vi "Initialization.vi"(3 "AdapterModuleRequired":bool=TRUE) -> (0 "InitDone":bool, 1 "IO Module ID":T1 {"InsertedIOModule ID" format="%x"; "Expected IO Module ID" format="%x"})   [LabVIEW 2013, in "IRIO.lvlib"]
uses:
  IRIO.lvlib
  <vilib>/eio/EIONode/EIONode.xnode
  <vilib>/rvi/eio/common/nirviEmuTemplateMethod_errors.vi
panel:
  out "IO Module IO Enabled":bool
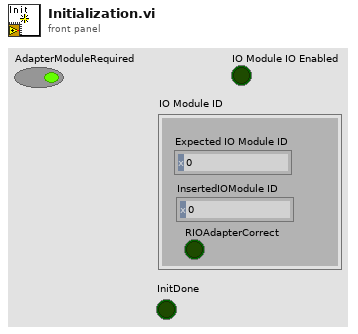
[diagram p1: front panel]
types:
  T1 = cluster{"Expected IO Module ID":u32, "InsertedIOModule ID":u32, "RIOAdapterCorrect":bool}
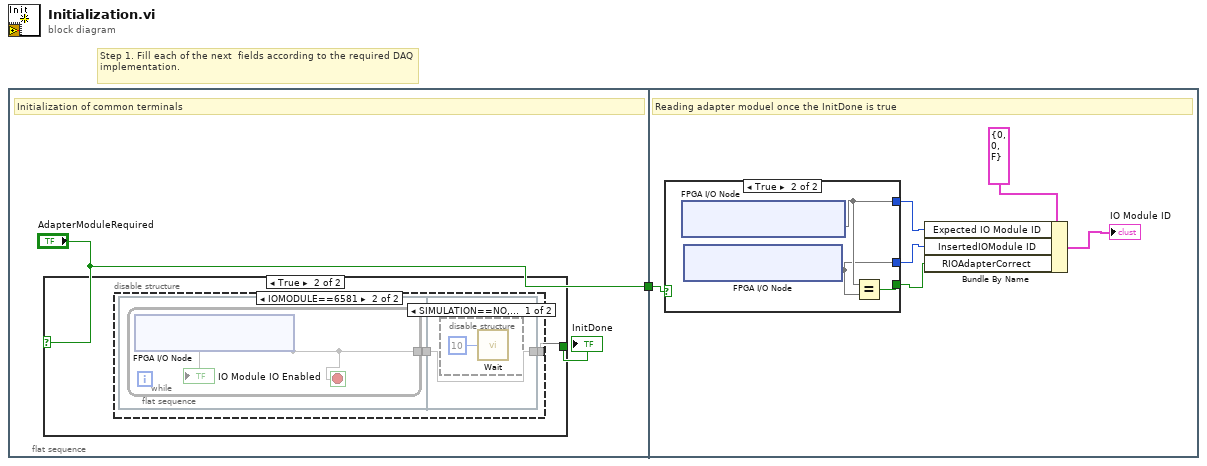
[diagram p0: block diagram]
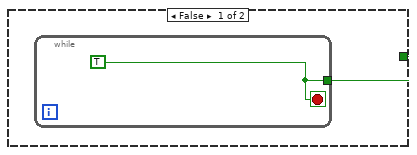
[diagram p2: hidden frame]
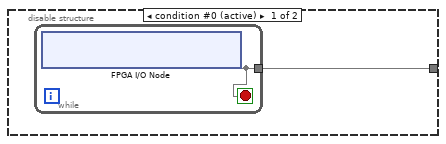
[diagram p3: hidden frame]
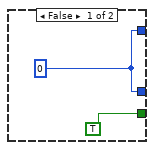
[diagram p5: hidden frame]
diagram:
  # "Step 1. Fill each of the next  fields according to the required DAQ implementation."
  n1 = flat-sequence {
    tunnel: ["AdapterModuleRequired"] -> w1
    tunnel: w1 -> [w20]
    frame #0 {
      # "Initialization of common terminals"
      n2 = case shown="True" "AdapterModuleRequired" {
        tunnel: [w4 w6] -> w3
        frame False {
          n3 = while {
            tunnel: [w5] -> w4
            stop <- w5 stop-if-true
            w5 = TRUE
          }
        }
        frame True {
          n4 = disable-structure shown="IOMODULE==6581" {
            disable-tunnel: [w7 w10] -> w6
            frame condition #0 (active) {
              n5 = while {
                tunnel: [w8] -> w7
                stop <- w8 stop-if-true
                n6 = xnode "FPGA I/O Node"() -> ("IO Module\\Initialization Done"=w8)  [unwired: 1 in, 1 out]
              }
            }
            frame condition #1 {
              n7 = flat-sequence {
                tunnel: [w11] -> w9
                tunnel: [w13] -> w10
                tunnel: w9 -> [w13]
                frame #0 {
                  n8 = while {
                    tunnel: [w12] -> w11
                    stop <- w12 stop-if-true
                    n9 = xnode "FPGA I/O Node"() -> ("IO Module IO Enabled"=w12)  [unwired: 1 in, 1 out]
                    "IO Module IO Enabled" <- w12
                  }
                }
                frame #1 {
                  n10 = disable-structure shown="SIMULATION==NO, Default" {
                    frame condition #0 (active) {
                      n11 = call "Wait"("Count(mSec)"=u32 10) -> ()  [unwired: 1 out]
                    }
                    frame condition #1 {
                    }
                  }
                }
              }
            }
          }
        }
      }
      "InitDone" <- w3
    }
    frame #1 {
      # "Reading adapter moduel once the InitDone is true"
      n12 = case shown="True" w20 {
        tunnel: [TRUE w25] -> w16
        tunnel: [w22 w24] -> w18
        tunnel: [w22 w23] -> w17
        frame False {
          w22 = u32 0
        }
        frame True {
          n13 = xnode "FPGA I/O Node"() -> ("Expected IO Module ID"=w24)  [unwired: 1 in, 1 out]
          n14 = xnode "FPGA I/O Node"() -> ("Inserted IO Module ID"=w23)  [unwired: 1 in, 1 out]
          n15 = Equal?(x=w24, y=w23) -> (x = y?=w25:bool)
        }
      }
      n16 = Bundle By Name(cluster=T1 {"Expected IO Module ID"=0, "InsertedIOModule ID"=0, "RIOAdapterCorrect"=FALSE} ("IO Module ID"), "Expected IO Module ID"=w18, "InsertedIOModule ID"=w17, "RIOAdapterCorrect"=w16) -> (→"IO Module ID":T1)
    }
  }
